vi "Save Text.vi"(8 "error in (no error)":errorcluster, 10 "Data":dbl, 11 "Text File in":refnum<class "Text File.lvclass">) -> (0 "error out":errorcluster, 3 "Text File out":refnum<class "Text File.lvclass">)   [LabVIEW 2020, in "Text File.lvlib" / "Text File.lvclass"]
uses:
  Text File.lvclass
  Text File.lvclass/Text File.ctl
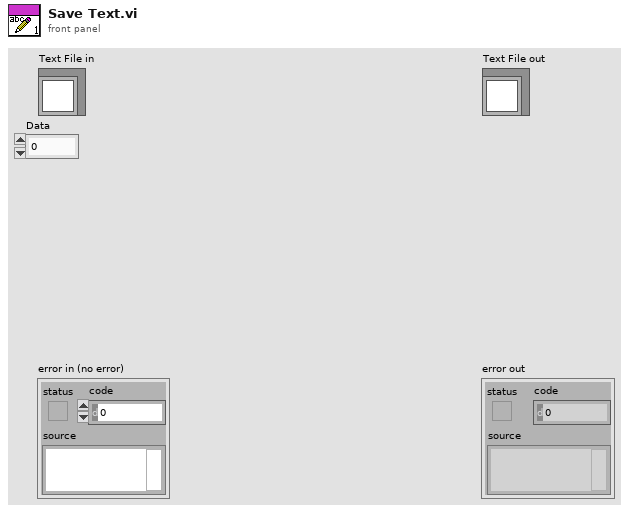
[diagram p1: front panel]
types:
  T1 = enum16{"open", "replace", "create", "open or create", "replace or create", "replace or create with confirmation"}
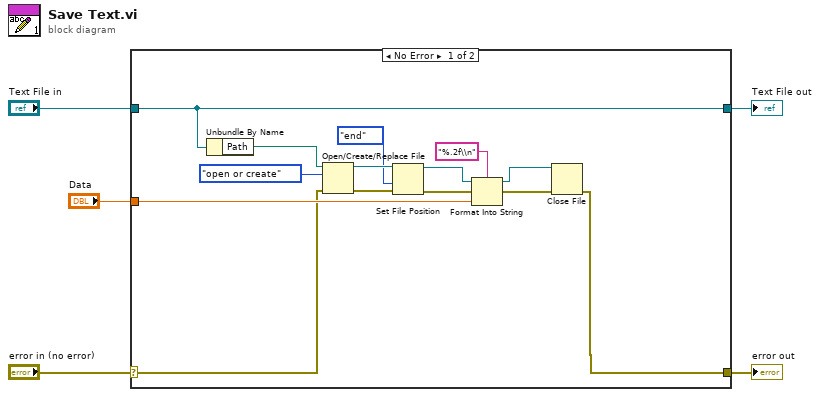
[diagram p0: block diagram]
diagram:
  n1 = case shown="No Error" "error in (no error)" {
    selector: "error in (no error)" -> [w7 w21]
    tunnel: [w6 w21] -> w4
    tunnel: [w9 w20] -> w2
    tunnel: "Text File in" -> [w9 w20]
    tunnel: "Data" -> [w8 _]
    frame No Error {
      n2 = Unbundle By Name(w9) -> ("Path"=w17:path)
      n3 = Open/Create/Replace File(file path (use dialog)=w17, error in=w7, operation (0:open)=T1."open or create") -> (refnum out=w18:refnum<file>, error out=w19:errorcluster)  [unwired: 3 in, 1 out]
      n4 = Set File Position(refnum=w18, from (0:start)=enum16{"start", "end", "current"}."end", error in=w19) -> (refnum out=w14:refnum<file>, error out=w15:errorcluster)  [unwired: 1 in]
      n5 = Format Into String(format string="%.2f\\n", initial string=w14, error in=w15, w8) -> (resulting string=w12:refnum<file>, error out=w13:errorcluster)
      n6 = Close File(refnum=w12, error in=w13) -> (error out=w6:errorcluster)  [unwired: 1 out]
    }
    frame Error {
    }
  }
  "error out" <- w4
  "Text File out" <- w2
